vi "Optimizer.vi"(11 "Optimize Parameters":T1={"Volt Step"={"X"=0.01, "Y"=0.01, "Z"=0.0}, "Num Iterations"=1, "Dwell Time (ms)"=100, "Volts Range"={"X"=0.1, "Y"=0.1, "Z"=0.0}, "Method"={"X"=enum."Max", "Y"=enum."Max", "Z"=enum."Max"}} {"Volts Range"."Z" min=0.0; "Volts Range"."Y" min=0.0; "Volts Range"."X" min=0.0; "Dwell Time (ms)" min=0; "Num Iterations" min=1 step=1; "Volt Step"."Z" min=1e-05; "Volt Step"."Y" min=1e-06; "Volt Step"."X" min=1e-06}) -> (3 "Final Counts/s":dbl)   [LabVIEW 2012]
uses:
  Strict Type Def - Optimize Parameters Cluster.ctl
  Channels.vi
  Global Vars.vi
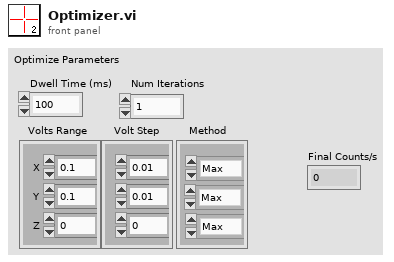
[diagram p1: front panel]
types:
  T1 = typedef "Strict Type Def - Optimize Parameters Cluster.ctl" = cluster{"Volt Step":cluster{"X":dbl, "Y":dbl, "Z":dbl}, "Num Iterations":i32, "Dwell Time (ms)":i32, "Volts Range":cluster{"X":dbl, "Y":dbl, "Z":dbl}, "Method":cluster{"X":enum16{"Max", "Gaussian"}, "Y":enum16{"Max", "Gaussian"}, "Z":enum16{"Max", "Gaussian"}}}
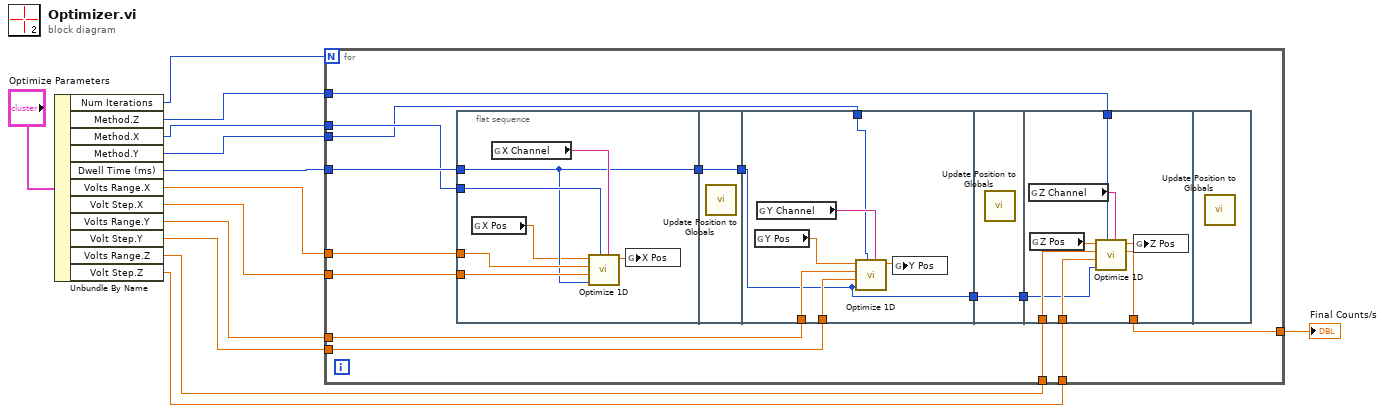
[diagram p0: block diagram]
diagram:
  n1 = Unbundle By Name("Optimize Parameters") -> ("Num Iterations"=w6:i32, "Method.Z"=w2:enum16{"Max", "Gaussian"}, "Method.X"=w3:enum16{"Max", "Gaussian"}, "Method.Y"=w11:enum16{"Max", "Gaussian"}, "Dwell Time (ms)"=w13:i32, "Volts Range.X"=w10:dbl, "Volt Step.X"=w9:dbl, "Volts Range.Y"=w8:dbl, "Volt Step.Y"=w7:dbl, "Volts Range.Z"=w5:dbl, "Volt Step.Z"=w4:dbl)
  n2 = for {
    N: w6 -> [_]
    tunnel: w13 -> [w28]
    tunnel: w3 -> [w25]
    tunnel: w11 -> [w24]
    tunnel: w10 -> [w23]
    tunnel: w9 -> [w22]
    tunnel: w8 -> [w21]
    tunnel: w7 -> [w20]
    tunnel: w5 -> [w19]
    tunnel: w4 -> [w18]
    tunnel: w2 -> [w15]
    tunnel: [w14] -> w1
    n3 = flat-sequence {
      tunnel: w28 -> [w30]
      tunnel: [w30] -> w27
      tunnel: w25 -> [w33]
      tunnel: w23 -> [w32]
      tunnel: w22 -> [w31]
      tunnel: w27 -> [w36]
      tunnel: [w36] -> w26
      tunnel: w26 -> [w37]
      tunnel: w24 -> [w41]
      tunnel: w21 -> [w39]
      tunnel: w20 -> [w38]
      tunnel: [w37] -> w16
      tunnel: [w44] -> w17
      tunnel: w16 -> [w44]
      tunnel: w19 -> [w50]
      tunnel: w18 -> [w49]
      tunnel: w17 -> [w48]
      tunnel: w15 -> [w47]
      tunnel: [w45] -> w14
      frame #0 {
        n4 = global read "Global Vars.vi" "X Pos"() -> (w29:dbl)
        n5 = global read "Channels.vi" "X Channel"() -> (w34:tag)
        n6 = call "Optimize 1D.vi"("AO Channel"=w34, "Fit Method"=w33, "Dwell Time (ms)"=w30, "Volt Step"=w31, "Volt Range"=w32, "Curr Pos"=w29) -> ("Final Pos"=w35:dbl)  [unwired: 4 in, 1 out]
        n7 = global write "Global Vars.vi" "X Pos"(w35) -> ()
      }
      frame #1 {
        n8 = call "Update Position to Globals.vi"() -> ()  [unwired: 11 in, 1 out]
      }
      frame #2 {
        n9 = global read "Global Vars.vi" "Y Pos"() -> (w40:dbl)
        n10 = global read "Channels.vi" "Y Channel"() -> (w43:tag)
        n11 = call "Optimize 1D.vi"("AO Channel"=w43, "Fit Method"=w41, "Dwell Time (ms)"=w37, "Volt Step"=w38, "Volt Range"=w39, "Curr Pos"=w40) -> ("Final Pos"=w42:dbl)  [unwired: 4 in, 1 out]
        n12 = global write "Global Vars.vi" "Y Pos"(w42) -> ()
      }
      frame #3 {
        n13 = call "Update Position to Globals.vi"() -> ()  [unwired: 11 in, 1 out]
      }
      frame #4 {
        n14 = global read "Channels.vi" "Z Channel"() -> (w52:tag)
        n15 = global read "Global Vars.vi" "Z Pos"() -> (w51:dbl)
        n16 = call "Optimize 1D.vi"("AO Channel"=w52, "Fit Method"=w47, "Dwell Time (ms)"=w48, "Volt Step"=w49, "Volt Range"=w50, "Curr Pos"=w51) -> ("Max Counts"=w45:dbl, "Final Pos"=w46:dbl)  [unwired: 4 in]
        n17 = global write "Global Vars.vi" "Z Pos"(w46) -> ()
      }
      frame #5 {
        n18 = call "Update Position to Globals.vi"() -> ()  [unwired: 11 in, 1 out]
      }
    }
  }
  "Final Counts/s" <- w1
